vi "CJ Processing.vi"() -> ()   [LabVIEW 2010]
uses:
  <vilib>/Utility/file.llb/Read From Spreadsheet File (string).vi
  <vilib>/Utility/file.llb/Write To Spreadsheet File (string).vi
panel:
  out "all rows 3":string[][](array[string])
  out "Array 3":string[](array[string])
  out "Effective Commission":dbl
  out "Effective Commission  Percentage":dbl[](array[numeric])
  out "Commission":dbl[](array[numeric])
  out "Commission/2":dbl[](array[numeric])
  out "Price":dbl[](array[numeric])
  out "Commisssion":string
  out "Array 2":string[](array[string])
  out "Array":dbl[](array[numeric])
  out "Effective Commission":dbl
  out "Effective Commission":dbl
  out "Comm / 2":dbl
  out "Half Commission":dbl
  out "Amazon Refined":string[][](array[string])
  out "2.5 Commission":dbl
  out "all rows 2":string[][](array[string])
  out "2.5 commission":dbl
  out "CJ Organized":string[][](array[string])
  out "ISBN 13":string
  out "extension":string
  out "SID":string
  out "Website Name":string
  out "Commission":string
  out "Price":string
  out "Date":string
  out "all rows":string[][](array[string])
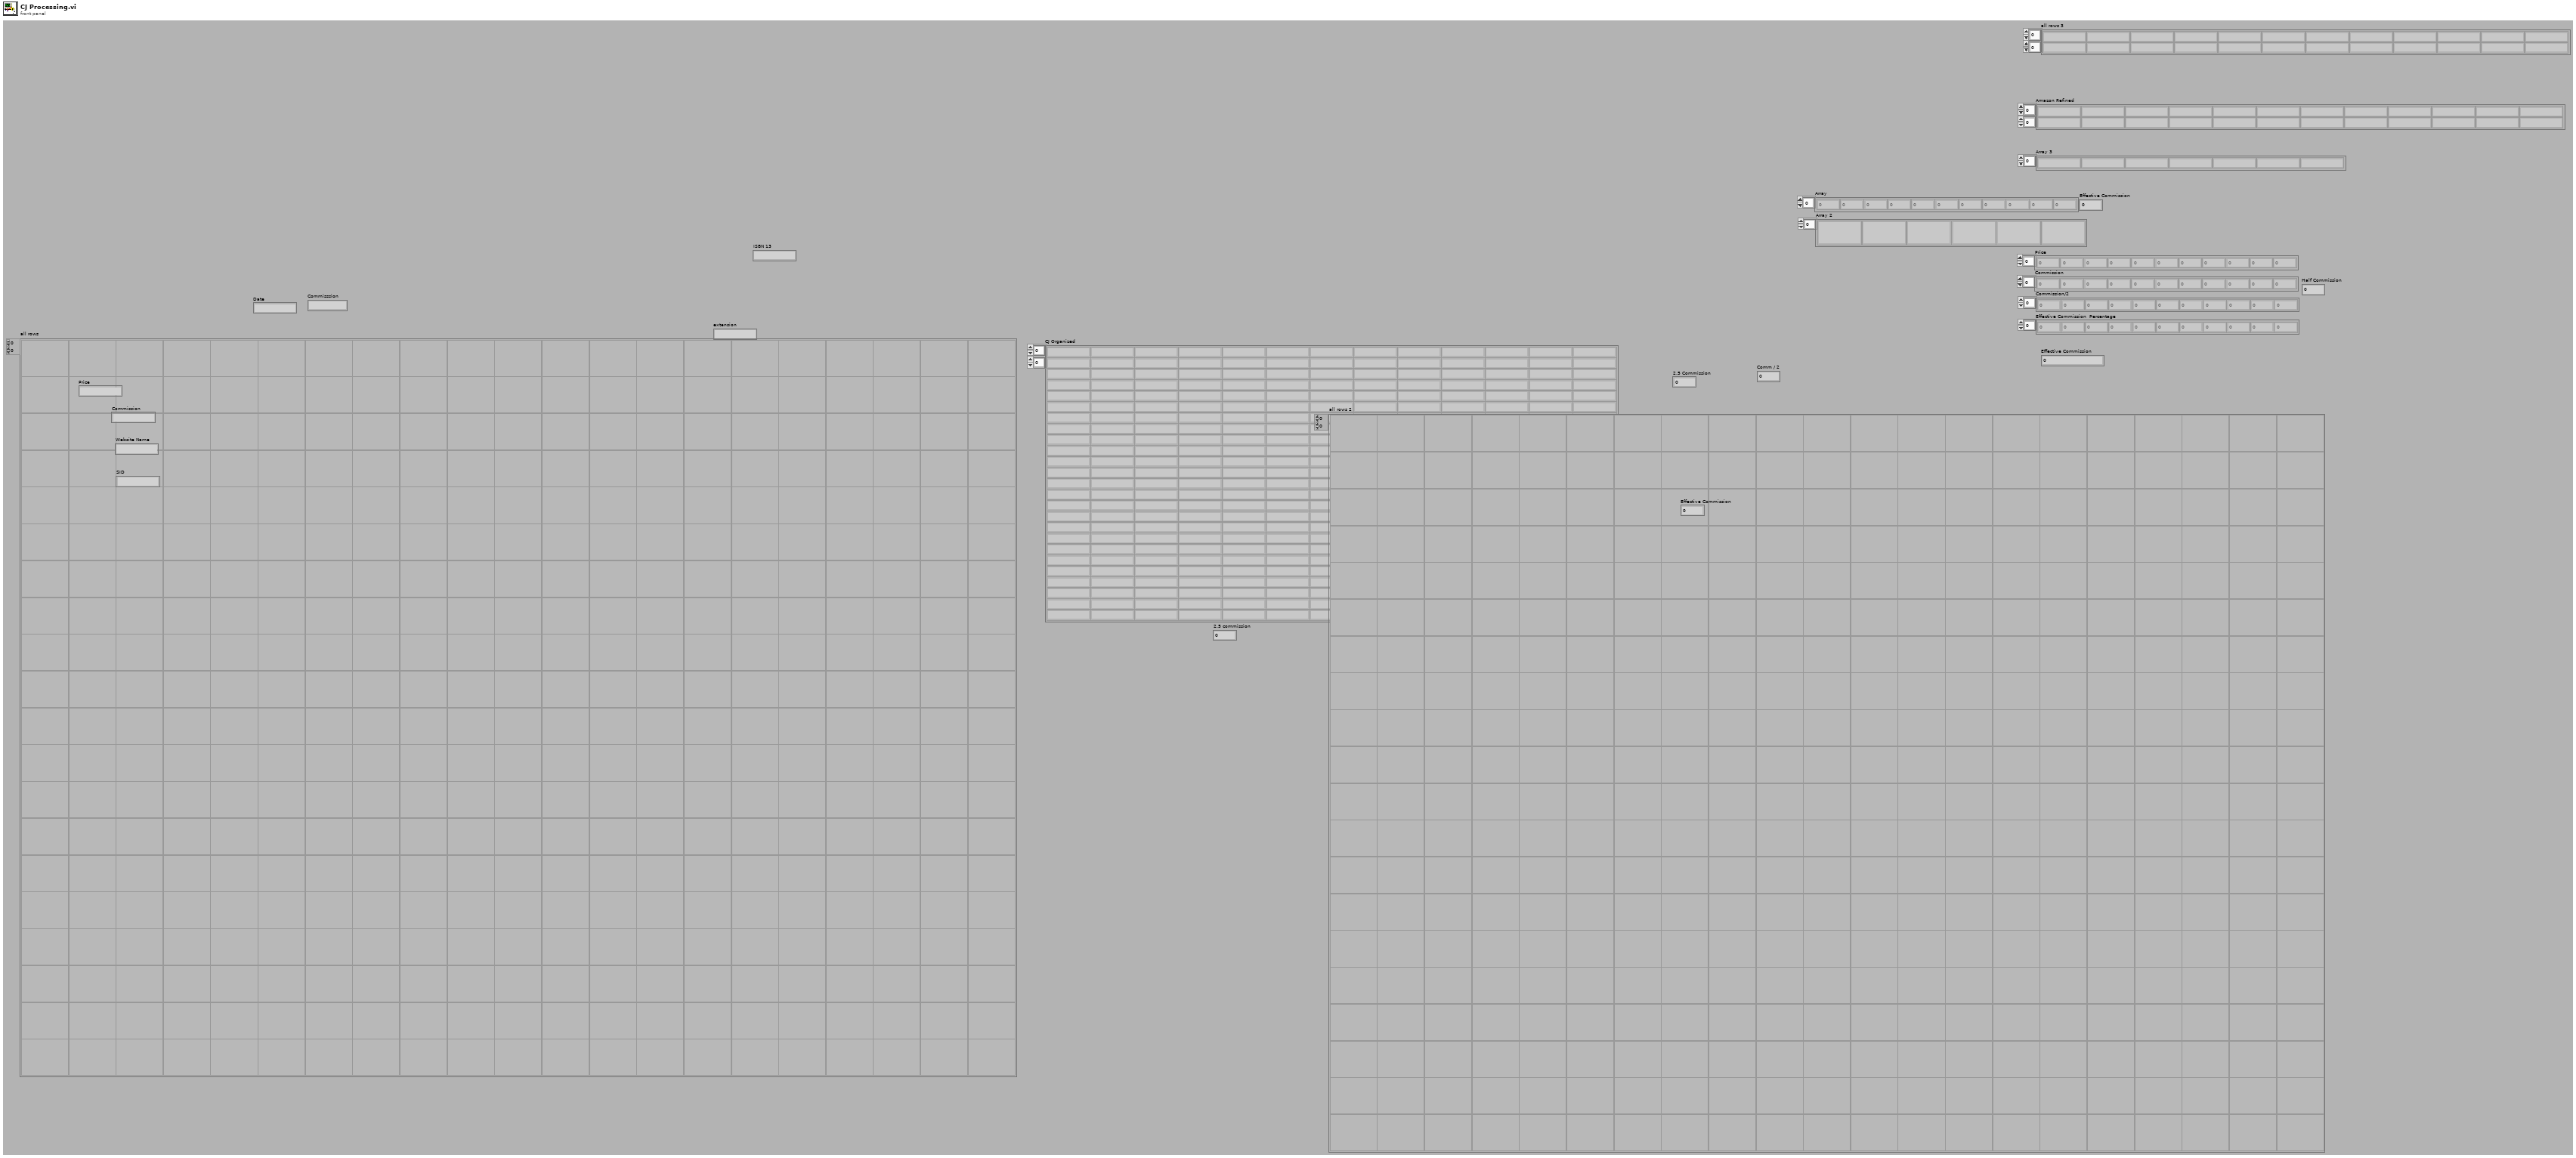
[diagram p1: front panel]
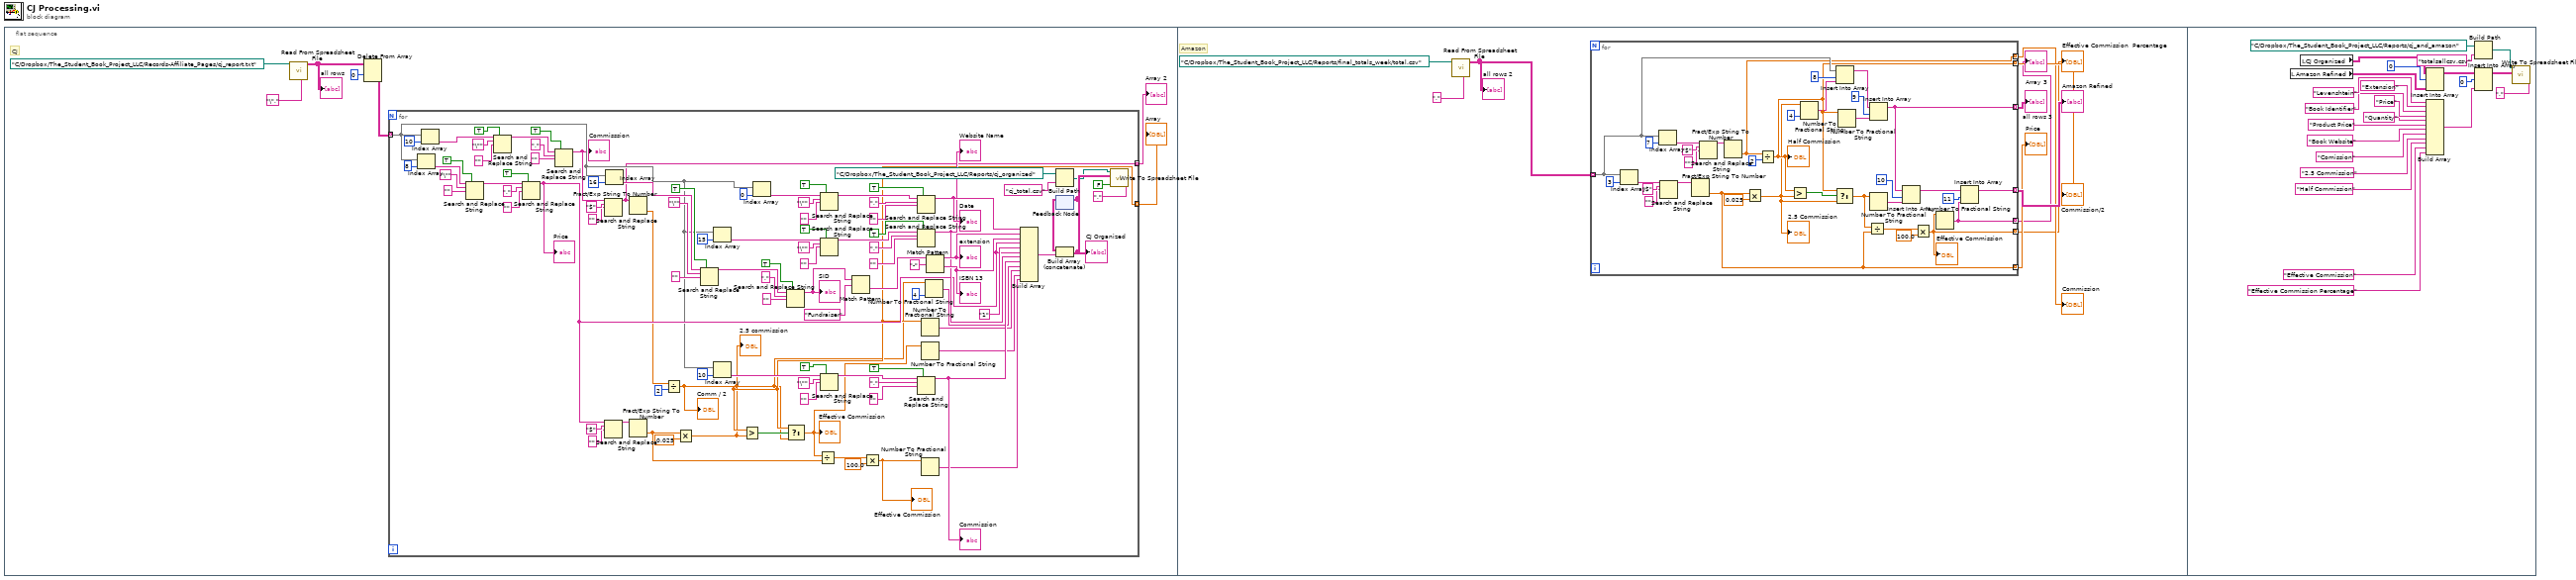
[diagram p0: block diagram]
diagram:
  n1 = flat-sequence {
    frame #0 {
      # "CJ"
      n2 = call-poly <vilib>:"Read From Spreadsheet File.vi"("delimiter (\\t)"="\"," ("delimiter (\\t)"), "file path (dialog if empty)"=path "C:/Dropbox/The_Student_Book_Project_LLC/Records-Affiliate_Pages/cj_report.txt" ("Directory Path to Start the Search")) -> ("all rows"=w5:string[][])  [unwired: 5 in, 4 out]
      "all rows" <- w5
      n3 = Delete From Array(array=w5, index (row)=0) -> (array with subset deleted=w3:string[][])  [unwired: 2 in, 1 out]
      n4 = for {
        tunnel: w3 -> [w29] mode=indexing
        tunnel: [w12] -> w2 mode=indexing
        tunnel: [w26] -> w1 mode=indexing
        n5 = Index Array(array=w29, index=8) -> (element=w96:string)
        n6 = Index Array(array=w29, index=10) -> (element=w18:string)
        n7 = Search and Replace String(replace all?=TRUE ("replace all? (F)"), input string=w96, search string="\"", replace string="" ("replace string (\"\")")) -> (result string=w91:string)  [unwired: 4 in, 3 out]
        n8 = Search and Replace String(replace all?=TRUE ("replace all? (F)"), input string=w18, search string="\"", replace string="" ("replace string (\"\")")) -> (result string=w21:string)  [unwired: 4 in, 3 out]
        n9 = Search and Replace String(replace all?=TRUE ("replace all? (F)"), input string=w91, search string=",", replace string="" ("replace string (\"\")")) -> (result string=w39:string)  [unwired: 4 in, 3 out]
        "Price" <- w39
        n10 = Search and Replace String(replace all?=TRUE ("replace all? (F)"), input string=w21, search string=",", replace string="" ("replace string (\"\")")) -> (result string=w17:string)  [unwired: 4 in, 3 out]
        "Commisssion" <- w17
        n11 = Search and Replace String(input string=w17, search string="$", replace string="" ("replace string (\"\")")) -> (result string=w26:string)  [unwired: 5 in, 3 out]
        n12 = Search and Replace String(input string=w39, search string="$", replace string="" ("replace string (\"\")")) -> (result string=w37:string)  [unwired: 5 in, 3 out]
        n13 = Index Array(array=w29, index=16) -> (element=w75:string)
        n14 = Fract/Exp String To Number(string=w26) -> (number=w33:dbl)  [unwired: 3 in, 1 out]
        n15 = Fract/Exp String To Number(string=w37) -> (number=w27:dbl)  [unwired: 3 in, 1 out]
        n16 = Divide(x=w33, y=2) -> (x/y=w12:dbl)
        "Comm / 2" <- w12
        n17 = Multiply(x=w27, y=0.025) -> (x*y=w11:dbl)
        "2.5 commission" <- w11
        n18 = Search and Replace String(replace all?=TRUE ("replace all? (F)"), input string=w75, search string="\"", replace string="" ("replace string (\"\")")) -> (result string=w70:string)  [unwired: 4 in, 3 out]
        n19 = Index Array(array=w29, index=15) -> (element=w82:string)
        n20 = Index Array(array=w29, index=10) -> (element=w89:string)
        n21 = Greater?(x=w12, y=w11) -> (0:w13:bool)
        n22 = Index Array(array=w29, index=0) -> (element=w103:string)
        n23 = Search and Replace String(replace all?=TRUE ("replace all? (F)"), input string=w70, search string=",", replace string="" ("replace string (\"\")")) -> (result string=w69:string)  [unwired: 4 in, 3 out]
        "SID" <- w69
        n24 = Select(t=w12, s=w13, f=w11) -> (s? t:f=w9:dbl)
        "Effective Commission" <- w9
        n25 = Divide(x=w9, y=w27) -> (x/y=w16:dbl)
        n26 = Search and Replace String(replace all?=TRUE ("replace all? (F)"), input string=w103, search string="\"", replace string="" ("replace string (\"\")")) -> (result string=w98:string)  [unwired: 4 in, 3 out]
        n27 = Search and Replace String(replace all?=TRUE ("replace all? (F)"), input string=w82, search string="\"", replace string="" ("replace string (\"\")")) -> (result string=w77:string)  [unwired: 4 in, 3 out]
        n28 = Search and Replace String(replace all?=TRUE ("replace all? (F)"), input string=w89, search string="\"", replace string="" ("replace string (\"\")")) -> (result string=w84:string)  [unwired: 4 in, 3 out]
        n29 = Match Pattern(string=w69, regular expression="Fundraiser") -> (after substring=w67:string)  [unwired: 1 in, 3 out]
        n30 = Multiply(x=w16, y=100.0) -> (x*y=w14:dbl)
        "Effective Commission" <- w14
        n31 = Search and Replace String(replace all?=TRUE ("replace all? (F)"), input string=w98, search string=",", replace string="" ("replace string (\"\")")) -> (result string=w65:string)  [unwired: 4 in, 3 out]
        "Date" <- w65
        n32 = Search and Replace String(replace all?=TRUE ("replace all? (F)"), input string=w77, search string=",", replace string="" ("replace string (\"\")")) -> (result string=w61:string)  [unwired: 4 in, 3 out]
        "Website Name" <- w61
        n33 = Search and Replace String(replace all?=TRUE ("replace all? (F)"), input string=w84, search string=",", replace string="" ("replace string (\"\")")) -> (result string=w60:string)  [unwired: 4 in, 3 out]
        "Commission" <- w60
        n34 = Number To Fractional String(number=w12) -> (F-format string=w28:string)  [unwired: 3 in]
        n35 = Number To Fractional String(number=w9) -> (F-format string=w8:string)  [unwired: 3 in]
        n36 = Number To Fractional String(number=w14) -> (F-format string=w10:string)  [unwired: 3 in]
        n37 = Number To Fractional String(number=w11, precision (6)=i16 4 ("width (-)")) -> (F-format string=w40:string)  [unwired: 2 in]
        n38 = Match Pattern(string=w67, regular expression="-") -> (before substring=w64:string, after substring=w63:string)  [unwired: 1 in, 2 out]
        "extension" <- w64
        "ISBN 13" <- w63
        n39 = Build Array(w65, w64, w63, w39, "1" ("element"), w39, w61, w60, w40, w28, w8, w10) -> (w59:string[])
        n40 = Build Path(base path=path "C:/Dropbox/The_Student_Book_Project_LLC/Reports/cj_organized" ("file path (dialog if empty)"), name or relative path="cj_total.csv") -> (appended path=w52:path)
        n41 = feedback #1() -> (w58:string[][])  [unwired: 1 in]
        n42 = Build Array (concatenate)(w58, w59) -> (w57:string[][])
        "CJ Organized" <- w57
        n43 = feedback-in #1(w57) -> ()
        n44 = call-poly <vilib>:"Write To Spreadsheet File.vi"("delimiter (\\t)"="," ("delimiter (\\t)"), "append to file? (new file:F)"=FALSE, "2D data"=w57, "file path (dialog if empty)"=w52) -> ()  [unwired: 4 in, 1 out]
      }
      "Array" <- w2
      "Array 2" <- w1
    }
    frame #1 {
      # "Amazon"
      n45 = call-poly <vilib>:"Read From Spreadsheet File.vi"("delimiter (\\t)"="," ("delimiter (\\t)"), "file path (dialog if empty)"=path "C:/Dropbox/The_Student_Book_Project_LLC/Reports/final_totals_week/total.csv" ("Directory Path to Start the Search")) -> ("all rows"=w112:string[][])  [unwired: 5 in, 4 out]
      "all rows 2" <- w112
      n46 = for {
        tunnel: w112 -> [w130] mode=indexing
        tunnel: [w115] -> w111 mode=indexing
        tunnel: [w119] -> w110 mode=indexing
        tunnel: [w122] -> w109 mode=indexing
        tunnel: [w129] -> w108 mode=indexing
        tunnel: [w126] -> w107 mode=indexing
        tunnel: [w118] -> w106 mode=indexing
        tunnel: [w117] -> w105 mode=indexing
        n47 = Index Array(array=w130, index=3) -> (element=w144:string)
        n48 = Index Array(array=w130, index=7) -> (element=w135:string)
        n49 = Search and Replace String(input string=w144, search string="$", replace string="" ("replace string (\"\")")) -> (result string=w146:string)  [unwired: 5 in, 3 out]
        n50 = Fract/Exp String To Number(string=w146) -> (number=w119:dbl)  [unwired: 3 in, 1 out]
        n51 = Search and Replace String(input string=w135, search string="$", replace string="" ("replace string (\"\")")) -> (result string=w137:string)  [unwired: 5 in, 3 out]
        n52 = Fract/Exp String To Number(string=w137) -> (number=w129:dbl)  [unwired: 3 in, 1 out]
        n53 = Multiply(x=w119, y=0.025) -> (x*y=w121:dbl)
        "2.5 Commission" <- w121
        n54 = Divide(x=w129, y=2) -> (x/y=w122:dbl)
        "Half Commission" <- w122
        n55 = Greater?(x=w122, y=w121) -> (0:w123:bool)
        n56 = Number To Fractional String(number=w121, precision (6)=i16 4 ("width (-)")) -> (F-format string=w143:string)  [unwired: 2 in]
        n57 = Insert Into Array(array=w130, index=8, new element=w143) -> (w132:string[])
        n58 = Select(t=w122, s=w123, f=w121) -> (s? t:f=w120:dbl)
        n59 = Number To Fractional String(number=w122) -> (F-format string=w134:string)  [unwired: 3 in]
        n60 = Divide(x=w120, y=w119) -> (x/y=w127:dbl)
        n61 = Insert Into Array(array=w132, index=9, new element=w134) -> (w117:string[])
        n62 = Number To Fractional String(number=w120) -> (F-format string=w124:string)  [unwired: 3 in]
        n63 = Insert Into Array(array=w117, index=10, new element=w124) -> (w116:string[])
        n64 = Multiply(x=w127, y=100.0) -> (x*y=w126:dbl)
        "Effective Commission" <- w126
        n65 = Number To Fractional String(number=w126) -> (F-format string=w118:string)  [unwired: 3 in]
        n66 = Insert Into Array(array=w116, index=11, new element=w118) -> (w115:string[])
      }
      "Amazon Refined" <- w111
      "Price" <- w110
      "Commission/2" <- w109
      "Commission" <- w108
      "Effective Commission  Percentage" <- w107
      "Array 3" <- w106
      "all rows 3" <- w105
    }
    frame #2 {
      n67 = local read "Amazon Refined"() -> (w166:string[][])
      n68 = local read "CJ Organized"() -> (w169:string[][])
      n69 = Insert Into Array(array=w169, index (row)=0, new element=w166) -> (w155:string[][])  [unwired: 1 in]
      n70 = Build Array("Levenshtein" ("name or relative path"), "Extension" ("element"), "Book Identifier" ("element"), "Price" ("element"), "Quantity" ("element"), "Product Price" ("element"), "Book Website" ("element"), "Comission" ("element"), "2.5 Commission" ("element"), "Half Commission" ("element"), "Effective Commission" ("element"), "Effective Commission Percentage" ("element")) -> (w154:string[])
      n71 = Build Path(base path=path "C:/Dropbox/The_Student_Book_Project_LLC/Reports/cj_and_amazon" ("file path (dialog if empty)"), name or relative path="totalsallcsv.csv") -> (appended path=w170:path)
      n72 = Insert Into Array(array=w155, index (row)=0, new element=w154) -> (w153:string[][])  [unwired: 1 in]
      n73 = call-poly <vilib>:"Write To Spreadsheet File.vi"("delimiter (\\t)"="," ("delimiter (\\t)"), "2D data"=w153, "file path (dialog if empty)"=w170) -> ()  [unwired: 5 in, 1 out]
    }
  }
